vi "Teleop.vi"(10 "Match Info":T1={"Autonomous Elapsed Seconds"=0.0, "TeleOp Elapsed Seconds"=0.0, "Disabled Elapsed Seconds"=0.0, "Visited Autonomous"=FALSE, "Visited TeleOp"=FALSE, "Visited Disabled"=FALSE, "Autonomous Settings"={"Autonomous Style"=enum."Independent", "VI Refnum"=refnum}}, 11 "Call Context":T2) -> ()   [LabVIEW 2012]
doc: "This VI is called for each TeleOp packet received from the DS where the robot is not disabled. It is often used to read from the joysticks and update I/O or to update setpoints for timed control loops. It should complete and return within 20 milliseconds or it may miss DS packets."
uses:
  <vilib>/Rock Robotics/WPI/DriverStation/WPI_DriverStationDerivedRobotMode.ctl
  <vilib>/Rock Robotics/WPI/DriverStation/WPI_DriverStationMatch Info.ctl
  Robot Global Data.vi
  <vilib>/Rock Robotics/WPI/Joystick/WPI_JoystickGetSetRefNum.vi
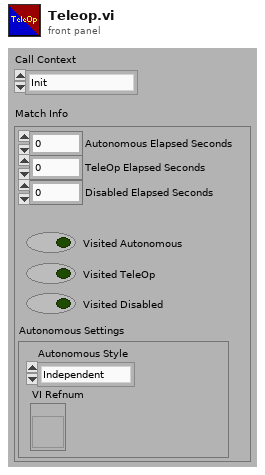
[diagram p1: front panel]
types:
  T1 = typedef "WPI_DriverStationMatch Info.ctl" = cluster{"Autonomous Elapsed Seconds":dbl, "TeleOp Elapsed Seconds":dbl, "Disabled Elapsed Seconds":dbl, "Visited Autonomous":bool, "Visited TeleOp":bool, "Visited Disabled":bool, "Autonomous Settings":cluster{"Autonomous Style":enum16{"Iterative", "Independent"}, "VI Refnum":refnum<vi>}}
  T2 = typedef "WPI_DriverStationDerivedRobotMode.ctl" = enum16{"Init", "Execute", "Stop"}
  T3 = typedef "WPI_JoystickDevRef.ctl" = cluster{"Device":T4}
  T4 = typedef "WPI_JoystickDeviceEnum.ctl" = enum16{"USB 1", "USB 2", "USB 3", "USB 4", "Kinect 1", "Kinect 2"}
  T5 = typedef "WPI_JoystickButtonState.ctl" = cluster{"Button 1":bool, "Button 2":bool, "Button 3":bool, "Button 4":bool, "Button 5":bool, "Button 6":bool, "Button 7":bool, "Button 8":bool, "Button 9":bool, "Button 10":bool, "Button 11":bool, "Button 12":bool}
  T6 = cluster{"axis 1 (x)":dbl, "axis 2 (y)":dbl, "axis 3 (throttle)":dbl, "axis 4":dbl, "axis 5":dbl, "axis 6":dbl}
  T7 = typedef "WPI_MotorControlDeviceRef.ctl" = cluster{"DeviceStatus":errorcluster, "Type":enum16{"PWM", "CAN"}, "PWM":cluster{"Digital Module":T8, "PWM Channel":T9, "DeadBand":T10}, "CAN":cluster{"Device Number":u8, "Control Mode":T11, "Semaphore":T12, "Max Vout":dbl}, "Invert":bool, "TransformRef":T13, "InvTransformRef":T13}
  T8 = typedef "FPGA_TypedefDigitalModule.ctl" = enum16{"Digital Module 1", "Digital Module 2"}
  T9 = typedef "FPGA_DIOPWMChannel.ctl" = enum8{"PWM 1", "PWM 2", "PWM 3", "PWM 4", "PWM 5", "PWM 6", "PWM 7", "PWM 8", "PWM 9", "PWM 10", "Invalid"}
  T10 = typedef "WPI_PWMDeadband.ctl" = cluster{"Name":string, "maxPositivePwm":i32, "minPositivePwm":i32, "centerPwm":i32, "maxNegativePwm":i32, "minNegativePwm":i32, "angularRange":u16}
  T11 = typedef "WPI_CANJaguar_ControlMode.ctl" = enum8{"Percent VBus", "Current", "Speed", "Position", "Voltage"}
  T12 = typedef "Semaphore RefNum" = refnum<k1>
  T13 = typedef "WPI_PWMTransform_ConPane.ctl" = refnum<vi>
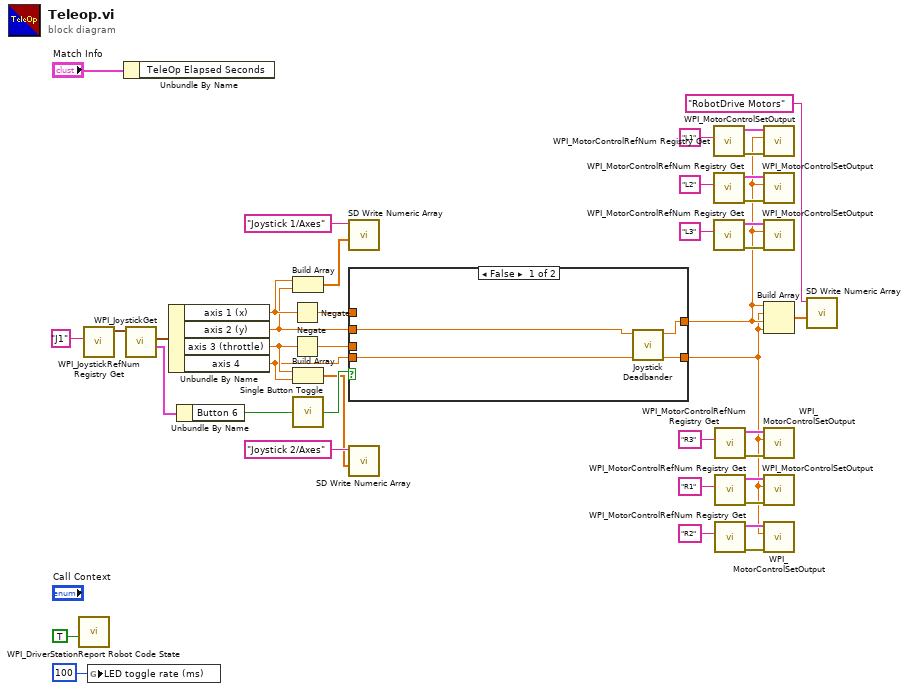
[diagram p0: block diagram]
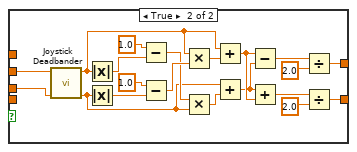
[diagram p2: hidden frame]
diagram:
  n1 = call <vilib>:"WPI_DriverStationReport Robot Code State.vi"("TeleOp"=TRUE ("Autonomous")) -> ()  [unwired: 10 in, 1 out]
  n2 = call <vilib>:"WPI_JoystickRefNum Registry Get.vi"("refnum name"="J1") -> ("JoystickDevRef"=w36:T3)  [unwired: 1 in, 9 out]
  n3 = global write "Robot Global Data.vi" "LED toggle rate (ms)"(u32 100 ("LED ms toggle rate")) -> ()
  n4 = Unbundle By Name("Match Info") -> ()  [unwired: 1 out]
  n5 = call <vilib>:"WPI_JoystickGet.vi"("JoystickDevRef"=w36) -> ("Buttons"=w14:T5, "Axes"=w35:T6)  [unwired: 1 in, 4 out]
  n6 = Unbundle By Name(w35) -> ("axis 1 (x)"=w5:dbl, "axis 2 (y)"=w4:dbl, "axis 3 (throttle)"=w2:dbl, "axis 4"=w1:dbl)
  n7 = Unbundle By Name(w14) -> ("Button 6"=w13:bool)
  n8 = Negate(x=w5) -> (-x=w10:dbl)
  n9 = Negate(x=w2) -> (-x=w9:dbl)
  n10 = Build Array(w5, w4) -> (w6:dbl[])
  n11 = Build Array(w2, w1) -> (w3:dbl[])
  n12 = call "Single Button Toggle.vi"("Input"=w13) -> ("Output"=w18:bool)
  n13 = call <vilib>:"SD Write Numeric Array.vi"("Numeric Array"=w6, "Name"="Joystick 1/Axes") -> ()  [unwired: 8 in, 2 out]
  n14 = case shown="False" w18 {
    tunnel: w4 -> [w45 w49]
    tunnel: w9 -> [_ w47]
    tunnel: w10 -> [_ _]
    tunnel: [w44 w51] -> w12
    tunnel: [w43 w50] -> w11
    tunnel: w1 -> [w42 _]
    frame False {
      n15 = call "Joystick Deadbander.vi"("y"=w42, "x"=w45) -> ("y edited"=w43:dbl, "X edited"=w44:dbl)  [unwired: 8 in]
    }
    frame True {
      n16 = call "Joystick Deadbander.vi"("y"=w47, "x"=w49) -> ("y edited"=w46:dbl, "X edited"=w48:dbl)  [unwired: 8 in]
      n17 = Absolute Value(x=w48) -> (abs(x)=w52:dbl)
      n18 = Absolute Value(x=w46) -> (abs(x)=w53:dbl)
      n19 = Subtract(x=1.0, y=w52) -> (x-y=w60:dbl)
      n20 = Subtract(x=1.0, y=w53) -> (x-y=w63:dbl)
      n21 = Multiply(x=w48, y=w63) -> (x*y=w62:dbl)
      n22 = Multiply(x=w60, y=w46) -> (x*y=w61:dbl)
      n23 = Add(x=w48, y=w62) -> (x+y=w57:dbl)
      n24 = Add(x=w46, y=w61) -> (x+y=w56:dbl)
      n25 = Subtract(x=w57, y=w56) -> (x-y=w55:dbl)
      n26 = Add(x=w56, y=w57) -> (x+y=w59:dbl)
      n27 = Divide(x=w55, y=2.0) -> (x/y=w51:dbl)
      n28 = Divide(x=w59, y=2.0) -> (x/y=w50:dbl)
    }
  }
  n29 = call <vilib>:"SD Write Numeric Array.vi"("Numeric Array"=w3, "Name"="Joystick 2/Axes") -> ()  [unwired: 8 in, 2 out]
  n30 = call <vilib>:"WPI_MotorControlRefNum Registry Get.vi"("refnum name"="L1") -> ("error out"=w34:errorcluster, "MotorControlDevRef"=w33:T7)  [unwired: 9 in]
  n31 = call <vilib>:"WPI_MotorControlRefNum Registry Get.vi"("refnum name"="L2") -> ("error out"=w31:errorcluster, "MotorControlDevRef"=w30:T7)  [unwired: 9 in]
  n32 = call <vilib>:"WPI_MotorControlRefNum Registry Get.vi"("refnum name"="L3") -> ("error out"=w28:errorcluster, "MotorControlDevRef"=w15:T7)  [unwired: 9 in]
  n33 = call <vilib>:"WPI_MotorControlRefNum Registry Get.vi"("refnum name"="R3") -> ("error out"=w20:errorcluster, "MotorControlDevRef"=w16:T7)  [unwired: 9 in]
  n34 = call <vilib>:"WPI_MotorControlRefNum Registry Get.vi"("refnum name"="R1") -> ("error out"=w26:errorcluster, "MotorControlDevRef"=w25:T7)  [unwired: 9 in]
  n35 = call <vilib>:"WPI_MotorControlRefNum Registry Get.vi"("refnum name"="R2") -> ("error out"=w23:errorcluster, "MotorControlDevRef"=w22:T7)  [unwired: 9 in]
  n36 = call <vilib>:"WPI_MotorControlSetOutput.vi"("error in (no error)"=w34, "Output"=w12, "MotorControlDevRef"=w33) -> ()  [unwired: 6 in, 3 out]
  n37 = call <vilib>:"WPI_MotorControlSetOutput.vi"("error in (no error)"=w31, "Output"=w12, "MotorControlDevRef"=w30) -> ()  [unwired: 6 in, 3 out]
  n38 = call <vilib>:"WPI_MotorControlSetOutput.vi"("error in (no error)"=w28, "Output"=w12, "MotorControlDevRef"=w15) -> ()  [unwired: 6 in, 3 out]
  n39 = Build Array(w12, w11, w12, w11) -> (w17:dbl[])
  n40 = call <vilib>:"WPI_MotorControlSetOutput.vi"("error in (no error)"=w20, "Output"=w11, "MotorControlDevRef"=w16) -> ()  [unwired: 6 in, 3 out]
  n41 = call <vilib>:"WPI_MotorControlSetOutput.vi"("error in (no error)"=w26, "Output"=w11, "MotorControlDevRef"=w25) -> ()  [unwired: 6 in, 3 out]
  n42 = call <vilib>:"WPI_MotorControlSetOutput.vi"("error in (no error)"=w23, "Output"=w11, "MotorControlDevRef"=w22) -> ()  [unwired: 6 in, 3 out]
  n43 = call <vilib>:"SD Write Numeric Array.vi"("Numeric Array"=w17, "Name"="RobotDrive Motors") -> ()  [unwired: 8 in, 2 out]
